vi "Show Or Hide Range.vi"(7 "Display State In":T1={"Current Channels Info"=[], "Help Prefix"="", "Max Display Size"=8, "Max Size"=8, "Show Buttons"=TRUE, "Data Valid"=refnum, "Show Range"=FALSE, "Range Items"=[], "Range Index"=[]} caption="State", 8 "error in (no error)":errorcluster, 10 "Panel":refnum<vi>, 11 "Channels Reference":refnum<vi>) -> (0 "error out":errorcluster)   [LabVIEW 2021, in "myRIO Channel List.xctl"]
uses:
  <vilib>/myRIO/Common/Express VI Framework/xctls/myRIO Channel List/myRIO Channel List.xctl
  <vilib>/myRIO/Common/Express VI Framework/xctls/myRIO Channel List/State.ctl
  <vilib>/myRIO/Common/Profile Manager Framework/typedefs/Channel Info.ctl
  <vilib>/myRIO/Common/Express VI Framework/typedefs/Data Validate Ref.ctl
  <vilib>/myRIO/Common/Express VI Framework/xctls/myRIO Channel List/typedefs/Channel View.ctl
  <vilib>/myRIO/Common/Express VI Framework/xctls/myRIO Channel List/typedefs/Error Icon.ctl
  <vilib>/myRIO/Common/Express VI Framework/xctls/myRIO Channel List/typedefs/Remove Channel.ctl
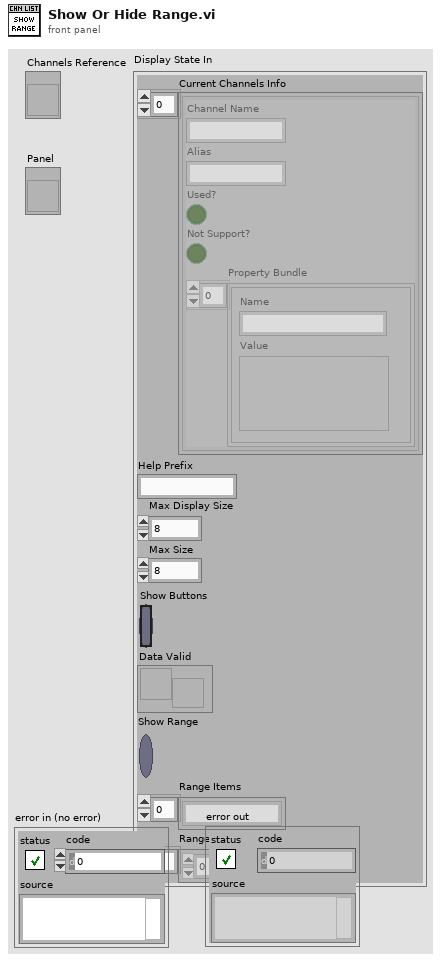
[diagram p1: front panel]
types:
  T1 = typedef "myRIO Channel List.xctl/State.ctl" = cluster{"Current Channels Info":T2[], "Help Prefix":string, "Max Display Size":i32, "Max Size":i32, "Show Buttons":bool, "Data Valid":T3, "Show Range":bool, "Range Items":string[], "Range Index":i32[]}
  T2 = typedef "Channel Info.ctl" = cluster{"Channel Name":string, "Alias":string, "Used?":bool, "Not Support?":bool, "Property Bundle":cluster{"Name":string, "Value":variant}[]}
  T3 = typedef "Data Validate Ref.ctl" = refnum<user-event>
  T4 = typedef "myRIO Channel List.xctl/Channel View.ctl" = cluster{"Error Icon":T5, "Channel Name":string, "Channel Alias":string, "Remove Channel":T6, "Index":i32, "Range":i32}
  T5 = typedef "myRIO Channel List.xctl/Error Icon.ctl" = bool
  T6 = typedef "myRIO Channel List.xctl/Remove Channel.ctl" = bool
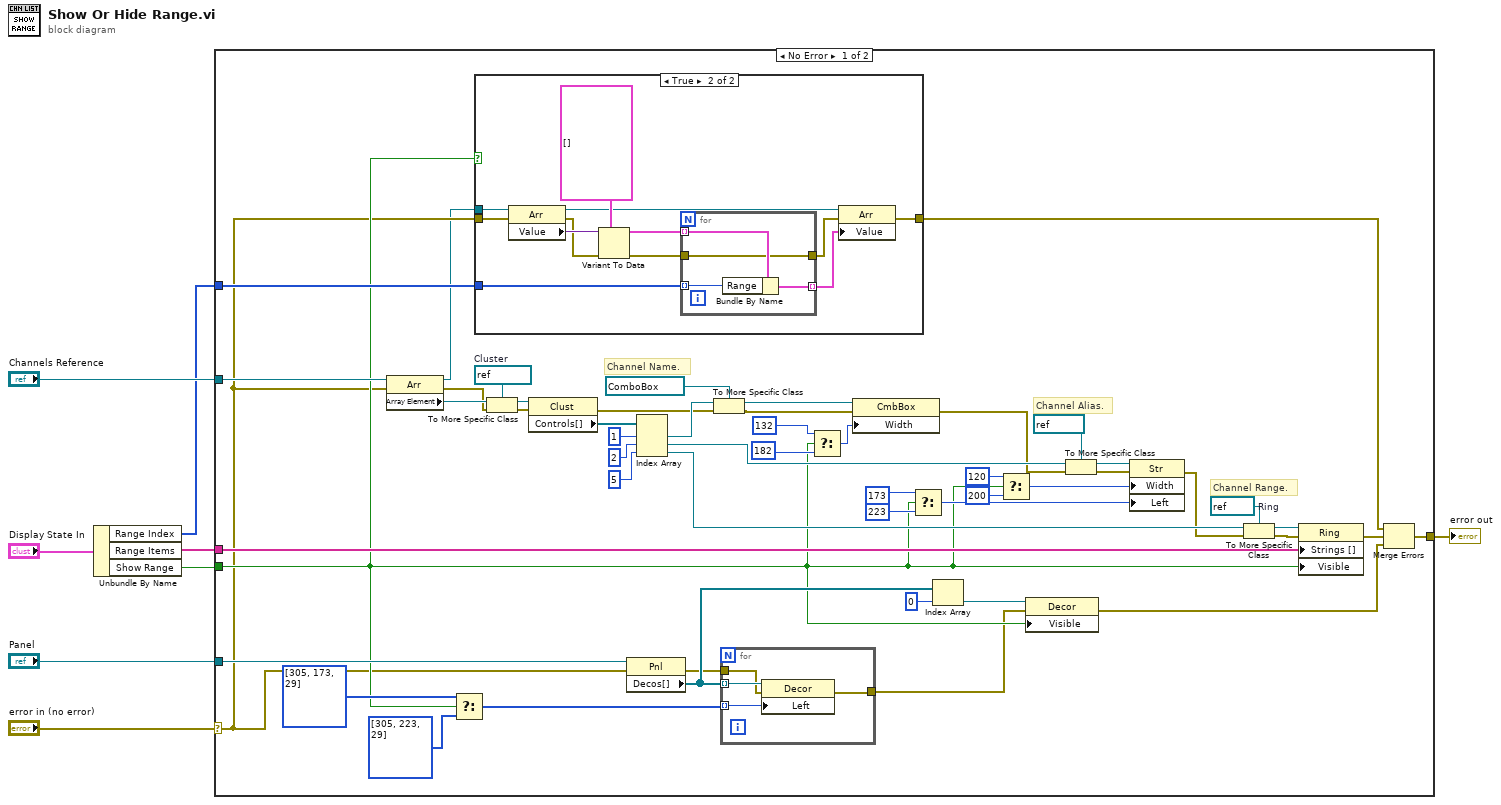
[diagram p0: block diagram]
diagram:
  n1 = Unbundle By Name("Display State In") -> ("Range Index"=w3:i32[], "Range Items"=w2:string[], "Show Range"=w6:bool)
  n2 = case shown="No Error" "error in (no error)" {
    selector: "error in (no error)" -> [w17 w82]
    tunnel: "Channels Reference" -> [w60 _]
    tunnel: w6 -> [w21 _]
    tunnel: "Panel" -> [w59 _]
    tunnel: w3 -> [w58 _]
    tunnel: w2 -> [w57 _]
    tunnel: [w11 w82] -> w1
    frame No Error {
      w40 = refnum<vi> refnum  # Ring
      w55 = refnum<vi> refnum  # Cluster
      # "Channel Range."
      # "Channel Alias."
      # "Channel Name."
      n3 = property class="Arr"(reference=w60, error in=w17) -> (reference out=w9:refnum<vi>, error out=w26:errorcluster, "Array Element"=w56:refnum<vi>)
      n4 = Select(t=i32[] [305, 173, 29], s=w21, f=i32[] [305, 223, 29]) -> (s? t:f=w35:i32[])
      n5 = case shown="True" w21 {
        tunnel: w9 -> [_ w73]
        tunnel: w58 -> [_ w72]
        tunnel: w17 -> [w61 w66]
        tunnel: [w61 w62] -> w12
        frame False {
        }
        frame True {
          n6 = property class="Arr"(reference=w73, error in=w66) -> (reference out=w69:refnum<vi>, error out=w65:errorcluster, "Value"=w71:variant)
          n7 = Variant To Data(error in=w65, type=T4[] [] ("Channels"), Variant=w71) -> (data=w68:T4[], error out=w64:errorcluster)
          n8 = for {
            tunnel: w68 -> [w77] mode=indexing
            tunnel: w72 -> [w76] mode=indexing
            tunnel: [w75] -> w67 mode=indexing
            tunnel: w64 -> [w74]
            tunnel: [w74] -> w63
            n9 = Bundle By Name(cluster=w77, "Range"=w76) -> (w75:T4)
          }
          n10 = property class="Arr"(reference=w69, error in=w63, "Value"=w67) -> (error out=w62:errorcluster)  [unwired: 1 out]
        }
      }
      n11 = To More Specific Class(target class=w55, reference=w56, error in=w26) -> (specific class reference=w54:refnum<vi>, error out=w25:errorcluster)
      n12 = property class="Clust"(reference=w54, error in=w25) -> (error out=w24:errorcluster, "Controls[]"=w53:refnum<vi>[])  [unwired: 1 out]
      n13 = property class="Pnl"(reference=w59, error in=w17) -> (error out=w16:errorcluster, "Decos[]"=w43:refnum<vi>[])  [unwired: 1 out]
      n14 = Index Array(array=w53, index #1=1 ("index"), index #2=2 ("index"), index #3=5 ("index")) -> (element #1=w49:refnum<vi>, element #2=w46:refnum<vi>, element #3=w39:refnum<vi>)
      n15 = To More Specific Class(target class=refnum<vi> refnum ("Combo Box"), reference=w49, error in=w24) -> (specific class reference=w48:refnum<vi>, error out=w23:errorcluster)
      n16 = for {
        tunnel: w43 -> [w81] mode=indexing
        tunnel: w35 -> [w80] mode=indexing
        tunnel: w16 -> [w79]
        tunnel: [w78] -> w15
        n17 = property class="Decor"(reference=w81, error in=w79, "Left"=w80) -> (error out=w78:errorcluster)  [unwired: 1 out]
      }
      n18 = Select(t=u32 132 ("Size:Width"), s=w21, f=u32 182 ("Size:Width")) -> (s? t:f=w10:u32)
      n19 = property class="CmbBox"(reference=w48, error in=w23, "Width"=w10) -> (error out=w22:errorcluster)  [unwired: 1 out]
      n20 = Select(t=173 ("Position:Left"), s=w21, f=223 ("Position:Left")) -> (s? t:f=w31:i32)
      n21 = Index Array(array=w43, index=0) -> (element=w41:refnum<vi>)
      n22 = Select(t=u32 120 ("Size:Width"), s=w21, f=u32 200 ("Size:Width")) -> (s? t:f=w32:u32)
      n23 = property class="Decor"(reference=w41, error in=w15, "Visible"=w21) -> (error out=w13:errorcluster)  [unwired: 1 out]
      n24 = To More Specific Class(target class=refnum<vi> refnum ("String"), reference=w46, error in=w22) -> (specific class reference=w44:refnum<vi>, error out=w20:errorcluster)
      n25 = property class="Str"(reference=w44, error in=w20, "Width"=w32, "Left"=w31) -> (error out=w19:errorcluster)  [unwired: 1 out]
      n26 = To More Specific Class(target class=w40, reference=w39, error in=w19) -> (specific class reference=w38:refnum<vi>, error out=w18:errorcluster)
      n27 = property class="Ring"(reference=w38, error in=w18, "Strings []"=w57, "Visible"=w21) -> (error out=w14:errorcluster)  [unwired: 1 out]
      n28 = Merge Errors(w12, w14, w13) -> (w11:errorcluster)
    }
    frame Error {
    }
  }
  "error out" <- w1
